vi "国际象棋双人.vi"() -> ()   [LabVIEW 2017]
panel:
  in  "数值":u8
  out "过程信息":string[](array[string])
  in  "请选择要变成的棋子":enum16{"士兵", "骑士", "主教", "战车", "皇后"}(ring)
  in  "新游戏":bool
  in  "Buttons":bool[][](array[boolean])=[[FALSE, FALSE, FALSE, FALSE, FALSE, FALSE, FALSE, FALSE], [FALSE, FALSE, FALSE, FALSE, FALSE, FALSE, FALSE, FALSE], [FALSE, FALSE, FALSE, FALSE, FALSE, FALSE, FALSE, FALSE], [FALSE, FALSE, FALSE, FALSE, FALSE, FALSE, FALSE, FALSE], [FALSE, FALSE, FALSE, FALSE, FALSE, FALSE, FALSE, FALSE], [FALSE, FALSE, FALSE, FALSE, FALSE, FALSE, FALSE, FALSE], [FALSE, FALSE, FALSE, FALSE, FALSE, FALSE, FALSE, FALSE], [FALSE, FALSE, FALSE, FALSE, FALSE, FALSE, FALSE, FALSE]]
  out "Indicator":bool[][](array[boolean])
  out "Y":i32
  out "X":i32
  in  "停止":bool
  out "移动方":enum16{"银色", "黑色"}(ring)
  out "棋盘":T1
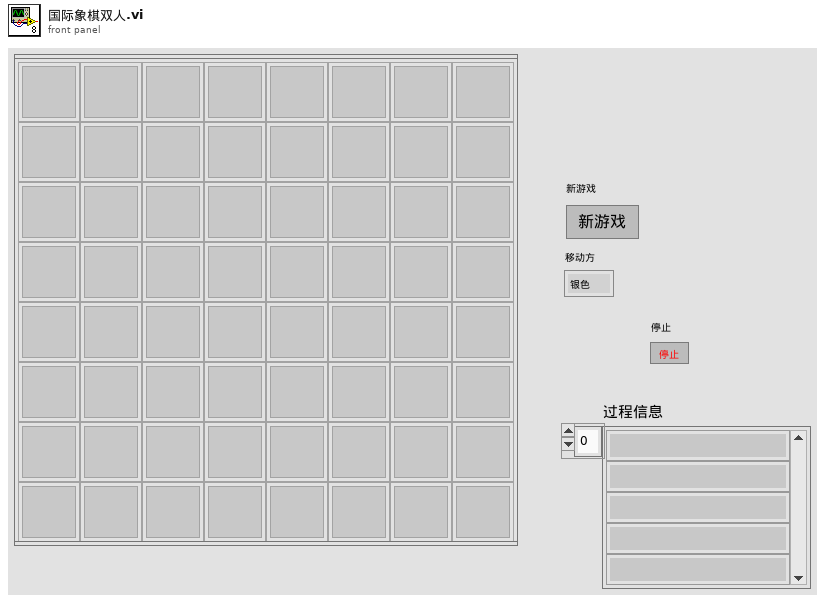
[diagram p1: front panel]
types:
  T1 = typedef "棋盘.ctl" = u16[][]
  T2 = cluster{"棋盘":u16[][], "银色棋子":cluster{"棋子类型":enum16{"士兵", "骑士", "主教", "战车", "皇后", "国王", "空"}, "X":u8, "Y":u8}[], "黑色棋子":cluster{"棋子类型":enum16{"士兵", "骑士", "主教", "战车", "皇后", "国王", "空"}, "X":u8, "Y":u8}[], "移动方":enum16{"银色", "黑色"}}
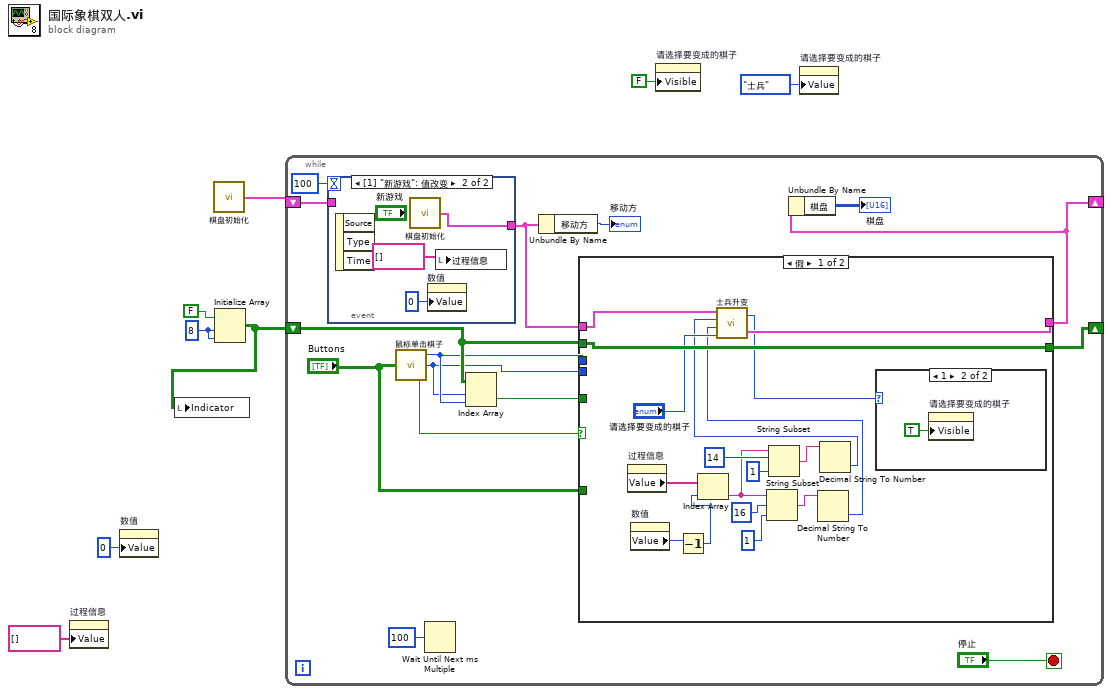
[diagram p0: block diagram]
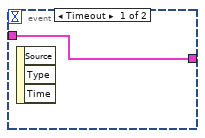
[diagram p2: hidden frame]
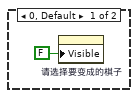
[diagram p3: hidden frame]
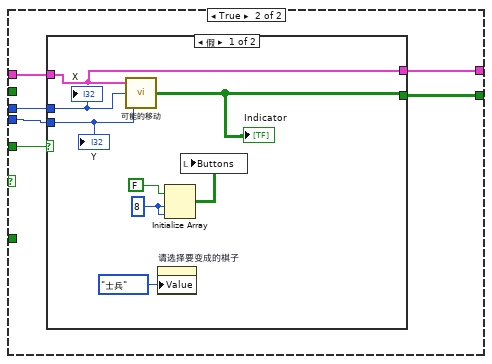
[diagram p4: hidden frame]
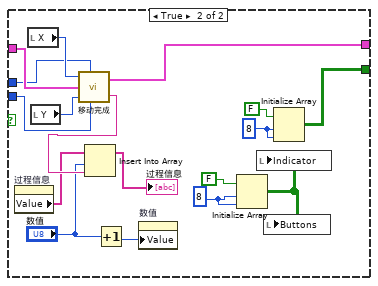
[diagram p5: hidden frame]
diagram:
  w7 = 8 ("维数大小")
  n1 = property on="过程信息" class="Arr (严格)"("Value"=string[] [] ("过程信息")) -> ()  [unwired: 2 in, 2 out]
  n2 = property on="数值" class="DigNum (严格)"("Value"=u8 0 ("数值")) -> ()  [unwired: 2 in, 2 out]
  n3 = call "棋盘初始化.vi"() -> ("游戏"=w8:T2)
  n4 = Initialize Array(FALSE, w7, w7) -> (w5:bool[][])
  n5 = local write "Indicator"(w5) -> ()
  n6 = while {
    shift-right: [w17] -> _
    shift-left: w8 -> [w12]
    shift-right: [w9] -> _
    shift-left: w5 -> [w22]
    stop <- "停止" stop-if-true
    n7 = event shown="[1] \"新游戏\": 值改变" {
      selector: _ -> [_ _]
      dyn-events: _ -> [_ _]
      timeout: 100 -> [_ _]
      tunnel: [w24 w27] -> w13
      tunnel: w12 -> [w24 _]
      event Timeout {
        n8 = event-data() -> ()  [unwired: 1 in, 3 out]
      }
      event "新游戏": Value Change {
        n9 = event-data() -> ()  [unwired: 1 in, 3 out]
        n10 = call "棋盘初始化.vi"() -> ("游戏"=w27:T2)
        n11 = property on="数值" class="DigNum (严格)"("Value"=u8 0 ("数值")) -> ()  [unwired: 2 in, 2 out]
        n12 = local write "过程信息"(string[] [] ("数组")) -> ()
      }
    }
    n13 = call "鼠标单击棋子.vi"("按钮"="Buttons") -> ("X"=w21:i32, "Y"=w20:i32, "是否单击"=w19:bool)
    n14 = Wait Until Next ms Multiple(millisecond multiple=u32 100 ("毫秒倍数")) -> ()  [unwired: 1 out]
    n15 = Index Array(array=w22, index (row)=w20, index (col)=w21) -> (element=w18:bool)
    n16 = Unbundle By Name(w13) -> ("移动方"=→"移动方":enum16{"银色", "黑色"})
    n17 = case shown="假" w19 {
      tunnel: w13 -> [w43 w49]
      tunnel: w22 -> [w44 _]
      tunnel: w21 -> [_ w52]
      tunnel: w20 -> [_ w51]
      tunnel: w18 -> [_ w50]
      tunnel: "Buttons" -> [_ _]
      tunnel: [w42 w48] -> w17
      tunnel: [w44 w47] -> w9
      frame False {
        n18 = property on="过程信息" class="Arr (严格)"() -> ("Value"=w40:string[])  [unwired: 2 in, 2 out]
        n19 = property on="数值" class="DigNum (严格)"() -> ("Value"=w39:u8)  [unwired: 2 in, 2 out]
        n20 = Decrement(x=w39) -> (x-1=w38:u8)
        n21 = Index Array(array=w40, index=w38) -> (element=w33:string)
        n22 = String Subset(string=w33, offset (0)=16 ("偏移量(0)"), length (rest)=1 ("长度（剩余）")) -> (substring=w30:string)
        n23 = String Subset(string=w33, offset (0)=14 ("偏移量(0)"), length (rest)=1 ("长度（剩余）")) -> (substring=w32:string)
        n24 = Decimal String To Number(string=w30) -> (number=w29:i32)  [unwired: 2 in, 1 out]
        n25 = Decimal String To Number(string=w32) -> (number=w31:i32)  [unwired: 2 in, 1 out]
        n26 = call "士兵升变.vi"("选项"="请选择要变成的棋子", "到达的Y"=w29, "到达的X"=w31, "输入的棋盘"=w43) -> ("输出棋盘"=w42:T2, "数值"=w28:u8)
        n27 = case shown="1" w28 {
          frame 0, Default {
            n28 = property on="请选择要变成的棋子" class="Enum (严格)"("Visible"=FALSE ("可见")) -> ()  [unwired: 2 in, 2 out]
          }
          frame 1 {
            n29 = property on="请选择要变成的棋子" class="Enum (严格)"("Visible"=TRUE ("可见")) -> ()  [unwired: 2 in, 2 out]
          }
        }
      }
      frame True {
        n30 = case shown="假" w50 {
          tunnel: w52 -> [w60 w68]
          tunnel: w51 -> [w59 w67]
          tunnel: w49 -> [w56 w77]
          tunnel: [w56 w66] -> w48
          tunnel: [w54 w74] -> w47
          frame False {
            w58 = 8 ("维数大小")
            n31 = call "可能的移动.vi"("Y"=w59, "X"=w60, "游戏"=w56) -> ("输出数组"=w54:bool[][])
            "Indicator" <- w54
            n32 = property on="请选择要变成的棋子" class="Enum (严格)"("Value"=enum16{"士兵", "骑士", "主教", "战车", "皇后"}."士兵" ("选项")) -> ()  [unwired: 2 in, 2 out]
            n33 = Initialize Array(FALSE, w58, w58) -> (w55:bool[][])
            n34 = local write "Buttons"(w55) -> ()
            "X" <- w60
            "Y" <- w59
          }
          frame True {
            w72 = 8 ("维数大小")
            w75 = 8 ("维数大小")
            n35 = property on="过程信息" class="Arr (严格)"() -> ("Value"=w61:string[])  [unwired: 2 in, 2 out]
            n36 = local read "X"() -> (w70:i32)
            n37 = local read "Y"() -> (w69:i32)
            n38 = call "移动完成.vi"("原始X"=w70, "移动后的X"=w68, "输入的棋盘"=w77, "原始Y"=w69, "移动后的Y"=w67) -> ("输出的棋盘"=w66:T2, "结果"=w65:string)
            n39 = Insert Into Array(array=w61, index="数值", new element=w65) -> (→"过程信息":string[])
            n40 = Increment(x="数值") -> (x+1=w63:u8)
            n41 = property on="数值" class="DigNum (严格)"("Value"=w63) -> ()  [unwired: 2 in, 2 out]
            n42 = Initialize Array(FALSE, w72, w72) -> (w71:bool[][])
            n43 = local write "Indicator"(w71) -> ()
            n44 = local write "Buttons"(w71) -> ()
            n45 = Initialize Array(FALSE, w75, w75) -> (w74:bool[][])
          }
        }
      }
    }
    n46 = Unbundle By Name(w17) -> ("棋盘"=→"棋盘":u16[][])
  }
  n47 = property on="请选择要变成的棋子" class="Enum (严格)"("Visible"=FALSE ("可见")) -> ()  [unwired: 2 in, 2 out]
  n48 = property on="请选择要变成的棋子" class="Enum (严格)"("Value"=enum16{"士兵", "骑士", "主教", "战车", "皇后"}."士兵" ("选项")) -> ()  [unwired: 2 in, 2 out]
